vi "Send Limit Current.vi"(8 "error in (no error)":errorcluster, 11 "57XX in":refnum<class "57XX.lvclass">) -> (0 "error out":errorcluster, 3 "57XX out":refnum<class "57XX.lvclass">)   [LabVIEW 2019, in "57XX.lvlib" / "57XX.lvclass"]
uses:
  Library/57XX.lvclass
  C:/Users/Public/Documents/Development/builds/Instruments/PowerSupply.lvlibp/Library/PowerSupply.lvclass
  Library/57XX.lvclass/57XX.ctl
  Accessors/Read Local Resource.vi
  Accessors/Write Local Resource.vi
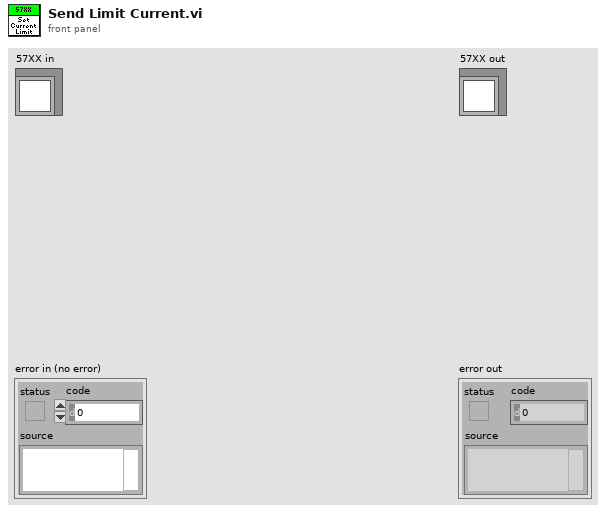
[diagram p1: front panel]
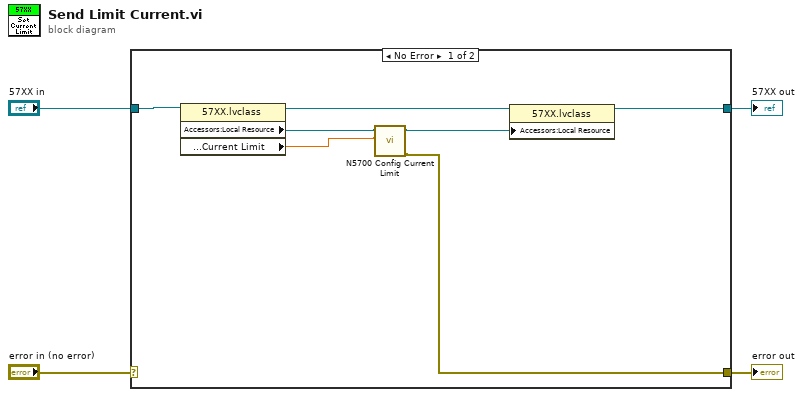
[diagram p0: block diagram]
diagram:
  n1 = case shown="No Error" "error in (no error)" {
    selector: "error in (no error)" -> [_ w13]
    tunnel: [w5 w13] -> w3
    tunnel: [w9 w12] -> w1
    tunnel: "57XX in" -> [w11 w12]
    frame No Error {
      n2 = property class="57XX.lvclass"(reference=w11) -> (reference out=w10:refnum<class "57XX.lvclass">, "Accessors:Local Resource"=w8:refnum<visa-resource-name>, "Accessors:Setting:Protection:Current Limit"=w6:dbl)  [unwired: 1 in, 1 out]
      n3 = call <instrlib>:"N5700 Config Current Limit.vi"("Current Limit"=w6, "VISA"=w8) -> ("error out"=w5:errorcluster, "VISA out"=w7:refnum<visa-resource-name>)  [unwired: 5 in]
      n4 = property class="57XX.lvclass"(reference=w10, "Accessors:Local Resource"=w7) -> (reference out=w9:refnum<class "57XX.lvclass">)  [unwired: 1 in, 1 out]
    }
    frame Error {
    }
  }
  "error out" <- w3
  "57XX out" <- w1
